vi "to string array.vi"(8 "error in (no error)":errorcluster, 11 "module configuration in":refnum<class "J1939 configuration.lvclass">) -> (0 "error out":errorcluster, 1 "Array":string[][](array[string]), 2 "version":string, 3 "module configuration out":refnum<class "J1939 configuration.lvclass">)   [LabVIEW 2017, in "J1939 configuration.lvclass"]
uses:
  J1939 configuration.lvclass
  J1939 configuration.lvclass/J1939 configuration.ctl
  <vilib>/NI/Tag Bus/tag/tag descriptor.lvclass/tag descriptor.ctl
  <vilib>/NI/Tag Bus Module Framework/channel/TBM channel.lvclass/TBM channel.ctl
  <vilib>/NI/Tag Bus Module Framework/channel/TBM channel.lvclass
  C:/Program Files (x86)/National Instruments/LabVIEW 2017/vi.lib/NI/Tag Bus/tag/tag descriptor.lvclass
  <vilib>/NI/Tag Bus/tag/tag descriptor.lvclass
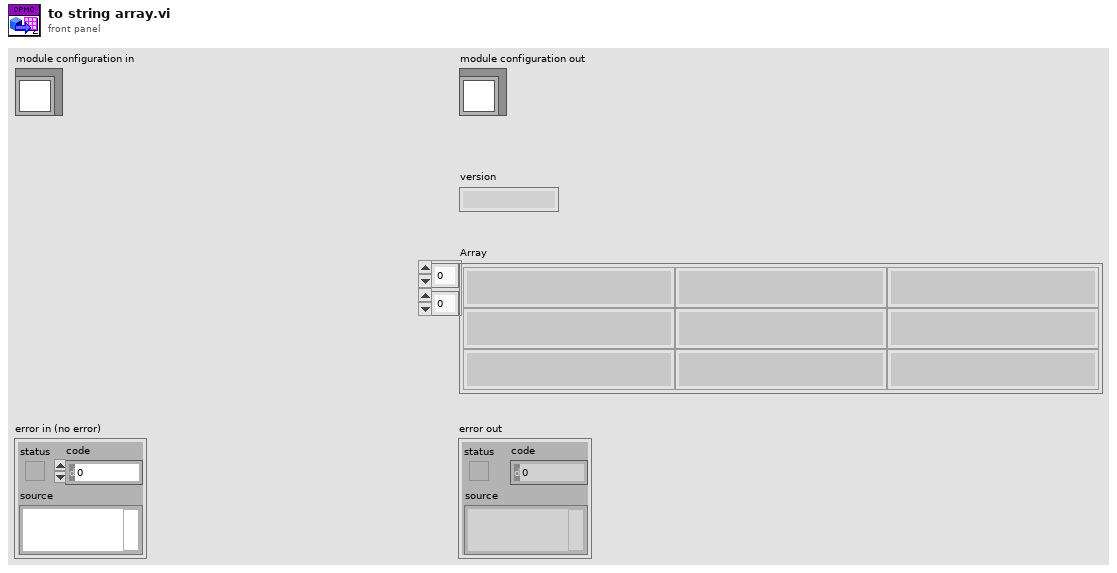
[diagram p1: front panel]
types:
  T1 = typedef "J1939 configuration.lvclass/Line.ctl" = cluster{"channel":refnum<class "TBM channel.lvclass">, "XNET Signal":refnum<k21>}
  T2 = typedef "tag bus.lvlib/tag descriptor.lvclass/Data Type.ctl" = enum16{"Double", "Single", "I64", "I32", "I16", "I8", "U64", "U32", "U16", "U8", "Boolean", "String", "Array of Double", "Array of Single", "Array of I64", "Array of I32", "Array of I16", "Array of I8", "Array of U64", "Array of U32", "Array of U16", "Array of U8", "Array of Boolean", "Array of String"}
  T3 = typedef "TBM channel.lvclass/channel classification.ctl" = enum16{"input data", "output data", "processing parameter", "processing result"}
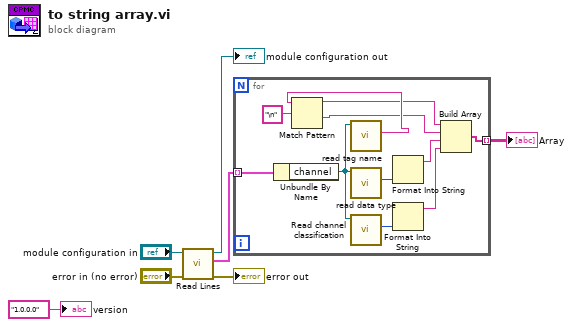
[diagram p0: block diagram]
diagram:
  n1 = call "Read Lines.vi"("error in (no error)"="error in (no error)", "J1939 configuration in"="module configuration in") -> ("error out"=→"error out":errorcluster, "Lines"=w5:T1[], "J1939 configuration out"=→"module configuration out":refnum<class "J1939 configuration.lvclass">)  [unwired: 7 in]
  n2 = for {
    tunnel: w5 -> [w18] mode=indexing
    tunnel: [w12] -> w1 mode=indexing
    n3 = Unbundle By Name(w18) -> ("channel"=w15:refnum<class "TBM channel.lvclass">)
    n4 = call <vilib>:"read tag name.vi"("system tag in"=w15) -> ("name"=w10:string)  [unwired: 8 in, 2 out]
    n5 = Match Pattern(string=w10, regular expression="\n" ("search string/char (-)")) -> (before substring=w9:string, after substring=w8:string)  [unwired: 1 in, 2 out]
    n6 = call <vilib>:"read data type.vi"("system tag in"=w15) -> ("data type"=w17:T2)  [unwired: 8 in, 2 out]
    n7 = call <vilib>:"Read channel classification.vi"("channel in"=w15) -> ("channel classification"=w14:T3)  [unwired: 8 in, 2 out]
    n8 = Format Into String(w17) -> (resulting string=w16:string)  [unwired: 3 in, 1 out]
    n9 = Format Into String(w14) -> (resulting string=w13:string)  [unwired: 3 in, 1 out]
    n10 = Build Array(w9, w8, w16, w13) -> (w12:string[])
  }
  "Array" <- w1
  "version" <- "1.0.0.0" ("version")
